vi "Main.vi"() -> ()   [LabVIEW 2019]
doc: "The myRIO Project template acquires acceleration data from the onboard accelerometer and displays the changes of acceleration values in a waveform chart."
uses:
  <vilib>/myRIO/Instrument Drivers/Onboard IO/PWM/typedefs/PWM Reference.ctl
  <vilib>/myRIO/Common/Instrument Driver Framework/Utilities/typedefs/myRIO Generic Hardware Reference.ctl
  <vilib>/myRIO/Common/Instrument Driver Framework/Utilities/typedefs/Hardware Version Enum.ctl
  <vilib>/myRIO/Common/Instrument Driver Framework/Utilities/typedefs/myRIO v1.0 Reference.ctl
  <vilib>/myRIO/Common/Instrument Driver Framework/Utilities/typedefs/Generic FPGA Reference.ctl
  <vilib>/myRIO/Common/Instrument Driver Framework/myRIO v1.0/PWM/typedefs/PWM Channels Enum.ctl
  <vilib>/myRIO/Instrument Drivers/Onboard IO/PWM/typedefs/PWM Configuration.ctl
  <vilib>/userDefined/High Color/nirio_resource_hc.ctl
  <vilib>/myRIO/Common/Instrument Driver Framework/Utilities/vis/Is FPGA Ref Available.vi
  <vilib>/myRIO/Common/Instrument Driver Framework/myRIO v1.0/PWM/vis/myRIO v1.1 Open PWM.vi
  <vilib>/myRIO/Instrument Drivers/Onboard IO/PWM/vis/Set Duty Cycle and Frequency.vi
  <vilib>/myRIO/Common/Instrument Driver Framework/Utilities/vis/Validate Channels.vi
  <vilib>/myRIO/Common/Instrument Driver Framework/myRIO v1.0/PWM/vis/myRIO v1.0 Reserve PWM.vi
  <vilib>/myRIO/Common/Instrument Driver Framework/myRIO v1.0/PWM/vis/myRIO v1.0 Build MUX Configuration PWM.vi
  <vilib>/myRIO/Common/Instrument Driver Framework/myRIO v1.0/Resource Manager/vis/myRIO v1.0 Reserve Channel List.vi
  <vilib>/myRIO/Common/Instrument Driver Framework/myRIO v1.0/Resource Manager/vis/myRIO v1.0 Create Configuration List.vi
  <vilib>/myRIO/Common/Instrument Driver Framework/myRIO v1.0/Resource Manager/vis/myRIO v1.0 Reserve Channel.vi
  <vilib>/myRIO/Common/Instrument Driver Framework/myRIO v1.0/Resource Manager/vis/myRIO v1.0 Unreserve Channel.vi
  <vilib>/myRIO/Common/Instrument Driver Framework/myRIO v1.0/Resource Manager/vis/myRIO v1.0 Build Mutex Name.vi
  <vilib>/Utility/VariantDataType/GetNumericInfo.vi
  <vilib>/Utility/error.llb/Error Cluster From Error Code.vi
  <vilib>/myRIO/Common/Instrument Driver Framework/myRIO v1.0/myRIO v1.1 Open.vi
  <vilib>/myRIO/Common/Instrument Driver Framework/Utilities/vis/IO Manager.vi
  <vilib>/myRIO/Common/Instrument Driver Framework/Utilities/vis/Configuration Manager.vi
  <vilib>/myRIO/Common/Instrument Driver Framework/myRIO v1.0/Resource Manager/vis/myRIO v1.0 Configure IO.vi
  <vilib>/myRIO/Common/Instrument Driver Framework/myRIO v1.0/myRIO v1.0 Close.vi
  <vilib>/myRIO/Common/Instrument Driver Framework/myRIO v1.0/PWM/vis/myRIO v1.0 Write PWM.vi
  <vilib>/myRIO/Express VI/Onboard IO/PWM/PWM Express VI.xnode
  <vilib>/myRIO/Instrument Drivers/Onboard IO/PWM/vis/myRIO PWM Open.xnode
  <vilib>/myRIO/Instrument Drivers/Onboard IO/PWM/PWM.lvlib
panel:
  in  "Numeric Control":i32
  in  "kruispunt verder":bool
  in  "hij mag weer verderrijden (na noodstop)":bool
  in  "noodstop":bool
  out "welk kruispunt":i32
  in  "Hoofdprogramma(einde)":bool
  out "de huidige afslag":string
  out "waardes van de reflectiesensor":dbl[](array[numeric])
  out "rechtermotor":dbl(knob) scale=0.0..10.0
  out "linkermotor":dbl(knob) scale=0.0..10.0
  in  "snelheidsverdeling":dbl(slide) scale=-5.0..5.0
  in  "snelheid":dbl(slide) scale=0.0..10.0
  in  "manual override?":bool
  in  "de afslagen":string[](array[string])
  # "links"
  # "rechts"
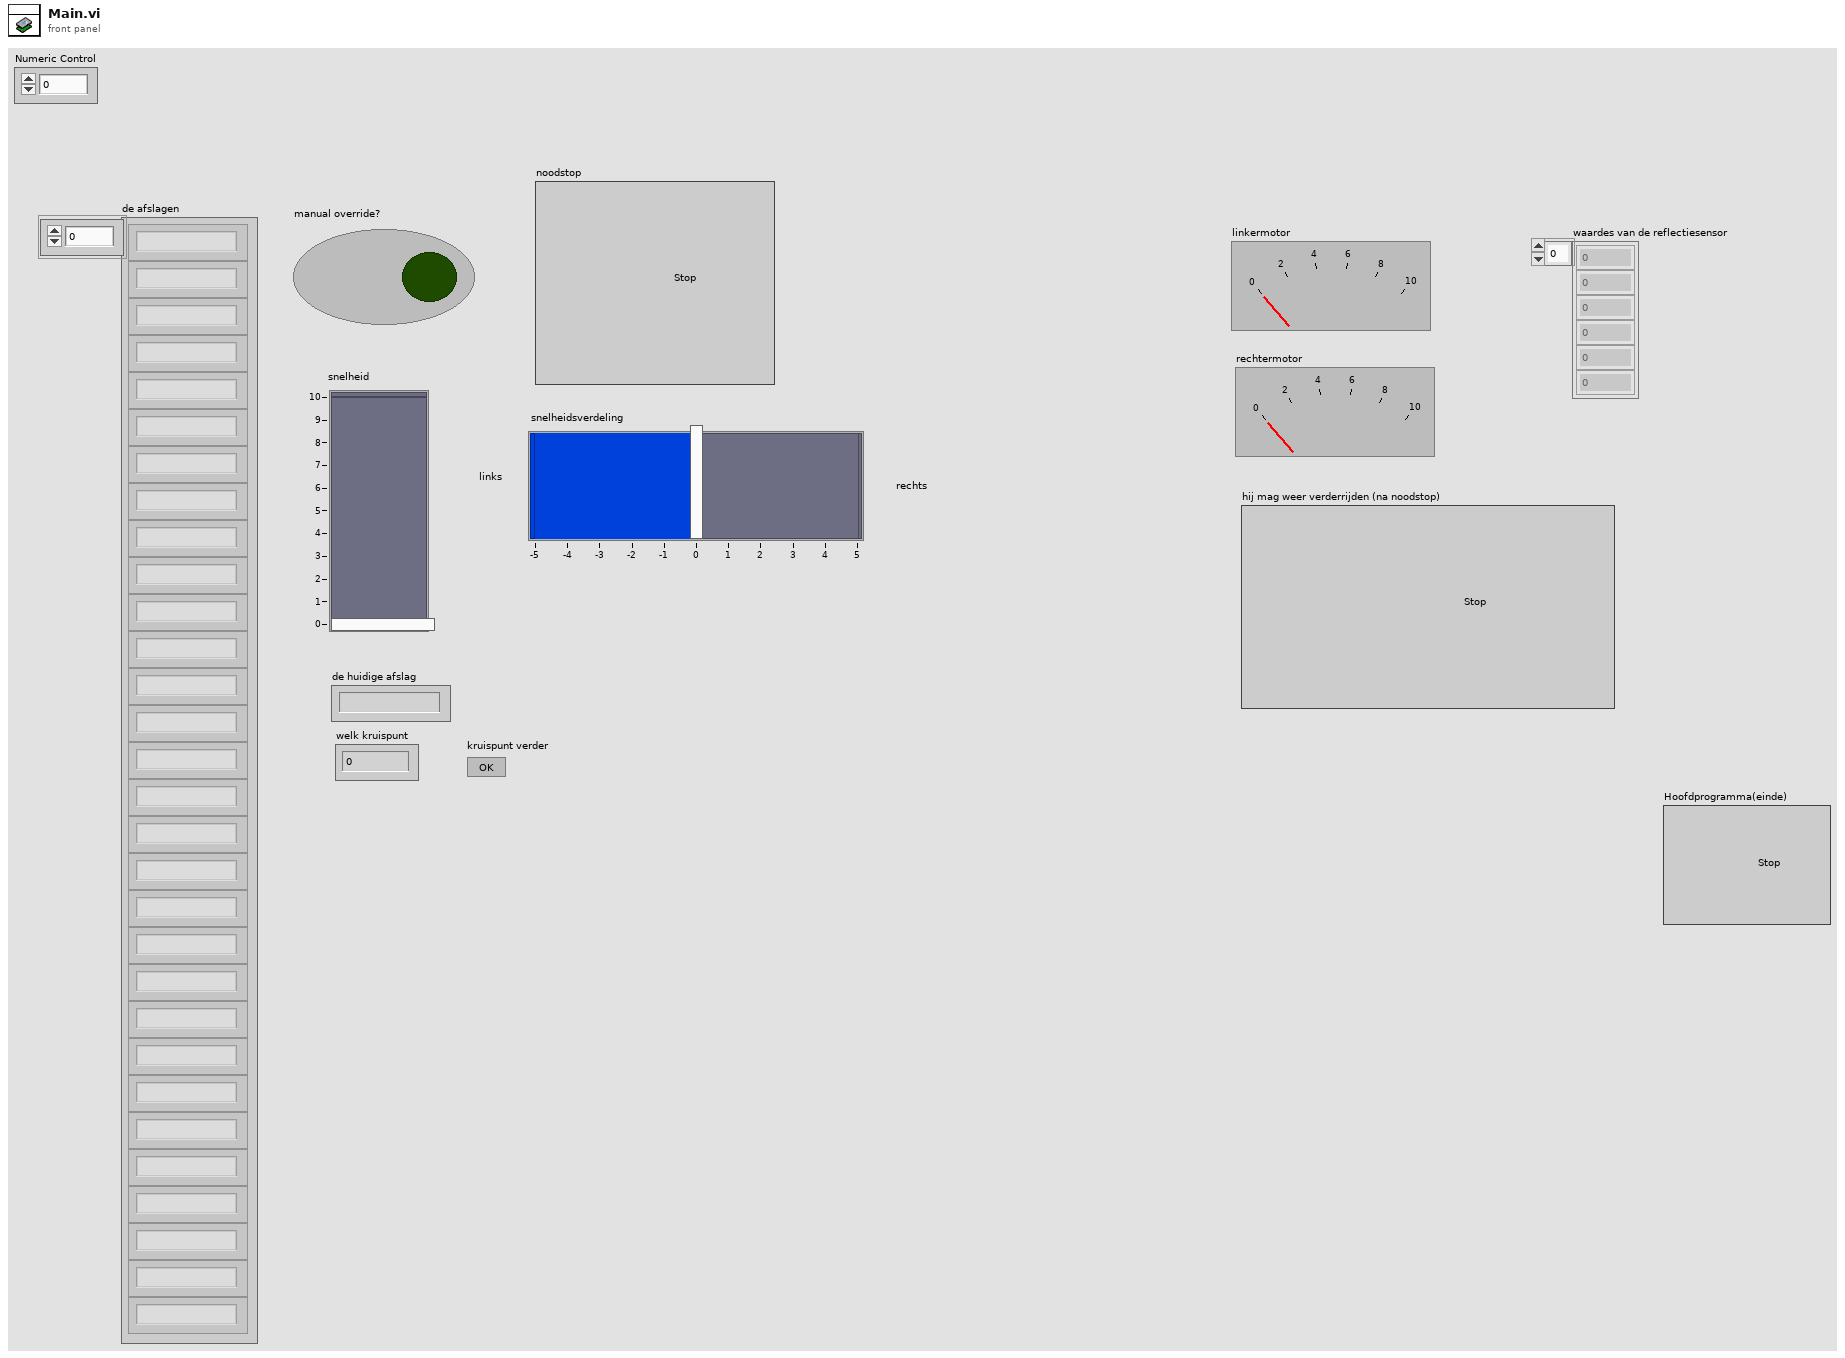
[diagram p1: front panel]
types:
  T1 = typedef "PWM.lvlib/PWM Reference.ctl" = cluster{"myRIO Reference":T2, "PWM Channels Enum":T6, "PWM Configuration":T7}
  T2 = typedef "myRIO Generic Hardware Reference.ctl" = cluster{"myRIO Model":T3, "myRIO Hardware Reference":T4}
  T3 = typedef "Hardware Version Enum.ctl" = enum16{"Unknown", "myRIO-1900", "myRIO-1950", "roboRIO", "NI ELVIS RIO CM", "ELVIS III"}
  T4 = typedef "myRIO v1.0 Reference.ctl" = cluster{"Generic FPGA Reference":T5, "Allow multiple opens":bool}
  T5 = typedef "Generic FPGA Reference.ctl" = refnum<k20>
  T6 = typedef "PWM Channels Enum.ctl" = enum16{"Not Connected", "C/PWM0", "C/PWM1", "A/PWM0", "A/PWM1", "A/PWM2", "A/PWM3", "A/PWM4", "A/PWM5", "A/PWM6", "A/PWM7", "A/PWM8", "A/PWM9", "A/PWM10", "A/PWM11", "A/PWM12", "A/PWM13", "A/PWM14", "A/PWM15", "A/PWM16", "A/PWM17", "A/PWM18", "A/PWM19", "B/PWM0", "B/PWM1", "B/PWM2", "B/PWM3", "B/PWM4", "B/PWM5", "B/PWM6", "B/PWM7", "B/PWM8", "B/PWM9", "B/PWM10", "B/PWM11", "B/PWM12", "B/PWM13", "B/PWM14", "B/PWM15", "B/PWM16", "B/PWM17", "B/PWM18", "B/PWM19", "PWM/PWM0", "PWM/PWM1", "PWM/PWM2", "PWM/PWM3", "PWM/PWM4", "PWM/PWM5", "PWM/PWM6", "PWM/PWM7", "PWM/PWM8", "PWM/PWM9"}
  T7 = typedef "PWM.lvlib/PWM Configuration.ctl" = cluster{"Frequency":dbl, "Duty Cycle":dbl}
  T8 = typedef "nirio_resource_hc.ctl" = tag
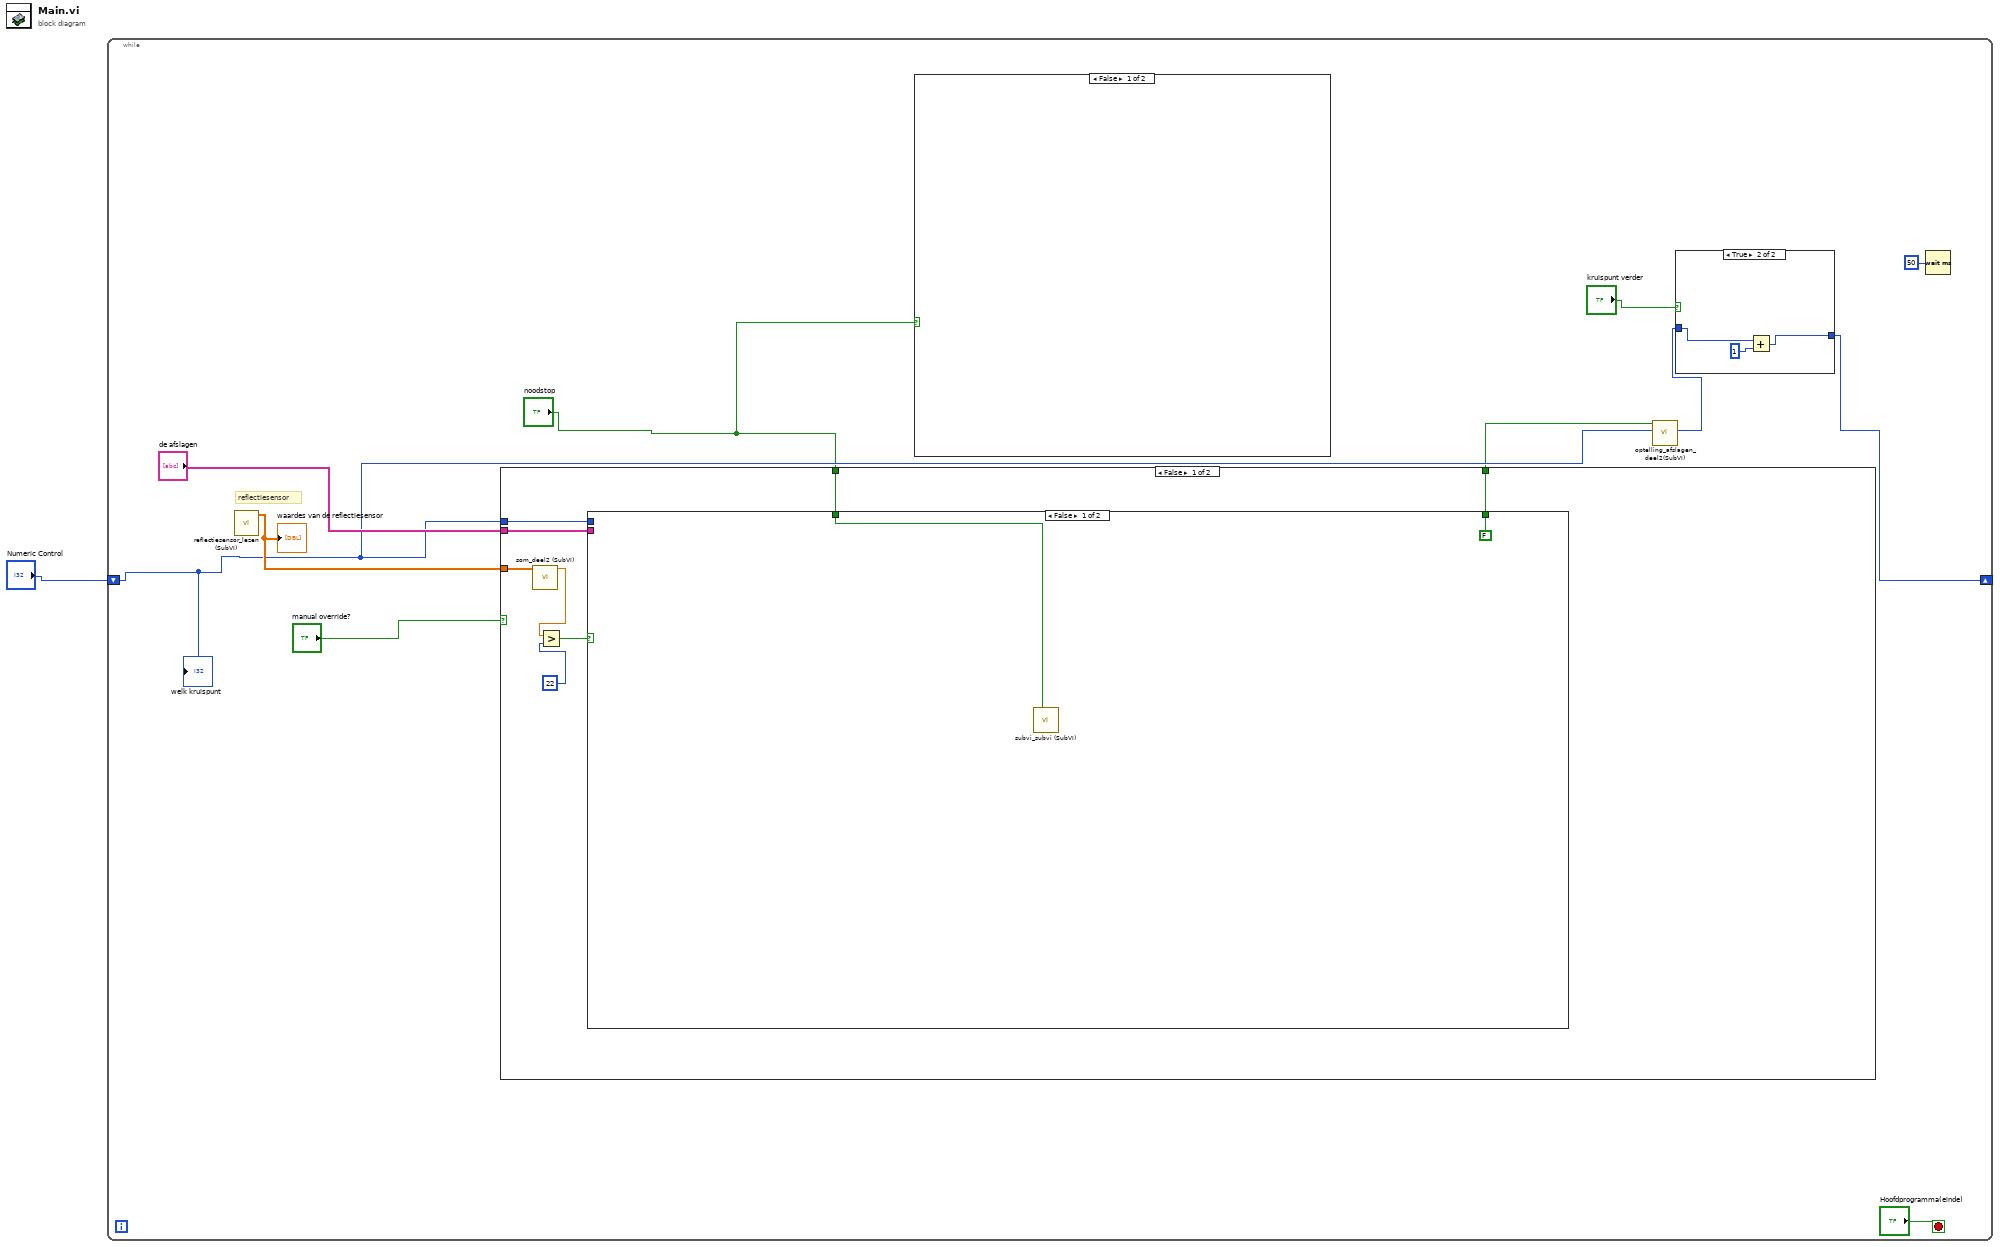
[diagram p0: block diagram]
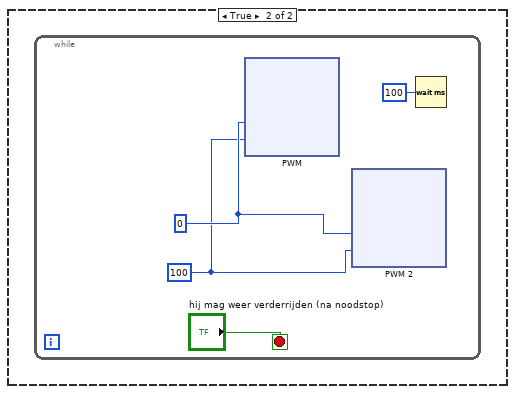
[diagram p3: hidden frame]
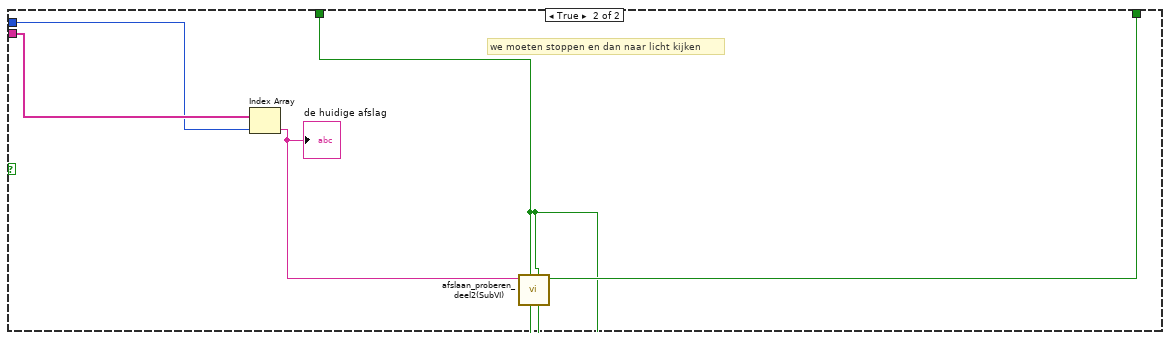
[diagram p4: hidden frame]
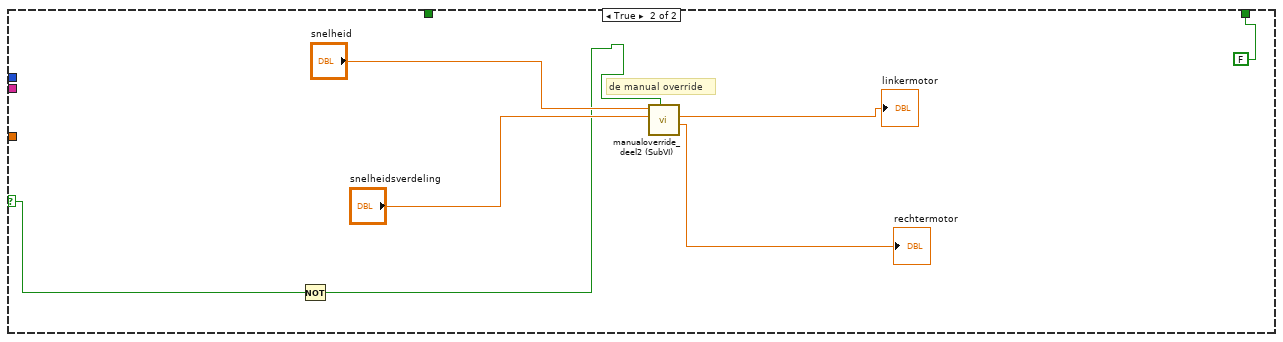
[diagram p5: hidden frame]
diagram:
  n1 = while {
    shift-right: [w4] -> _
    shift-left: "Numeric Control" -> [w9]
    stop <- "Hoofdprogramma(einde)" stop-if-true
    # "reflectiesensor"
    n2 = call "reflectiesensor_lezen (SubVI).vi"() -> ("Values"=w11:dbl[])  [unwired: 11 in]
    "waardes van de reflectiesensor" <- w11
    n3 = case shown="False" "manual override?" {
      selector: "manual override?" -> [_ w107]
      tunnel: w11 -> [w98 _]
      tunnel: "de afslagen" -> [w97 _]
      tunnel: w9 -> [w96 _]
      tunnel: [w92 FALSE] -> w8
      tunnel: "noodstop" -> [w91 _]
      frame False {
        n4 = call "som_deel2 (SubVI).vi"("array"=w98) -> ("x+y"=w95:dbl)  [unwired: 10 in]
        n5 = Greater?(x=w95, y=22) -> (0:w93:bool)
        n6 = case shown="False" w93 {
          tunnel: w97 -> [_ w105]
          tunnel: w96 -> [_ w104]
          tunnel: [FALSE w102] -> w92
          tunnel: w91 -> [w99 w101]
          frame False {
            n7 = call "subvi_subvi (SubVI).vi"("stop"=w99) -> ()  [unwired: 11 in]
          }
          frame True {
            # "we moeten stoppen en dan naar licht kijken"
            n8 = Index Array(array=w105, index=w104) -> (element=w103:string)
            "de huidige afslag" <- w103
            n9 = call "afslaan_proberen_deel2(SubVI).vi"("stop 3"=w101, "stop"=w101, "stop 2"=w101, "universele stop"=w101, "element"=w103) -> ("OK Button 2"=w102:bool)  [unwired: 6 in]
          }
        }
      }
      frame True {
        # "de manual override"
        n10 = Not(x=w107) -> (.not. x?=w106:bool)
        n11 = call "manualoverride_deel2 (SubVI).vi"("stop"=w106, "snelheidsverdeling"="snelheidsverdeling", "snelheid"="snelheid") -> ("rechtermotor na"=→"rechtermotor":dbl, "linkermotor na"=→"linkermotor":dbl)  [unwired: 7 in]
      }
    }
    n12 = case shown="False" "noodstop" {
      frame False {
      }
      frame True {
        n13 = while {
          stop <- "hij mag weer verderrijden (na noodstop)" stop-if-true
          w17 = 100
          w18 = 0
          n14 = xnode "PWM"("Duty Cycle"=w18, "Frequency [Hz]"=w17) -> ()  [unwired: 1 in, 1 out]
          n15 = xnode "PWM 2"("Duty Cycle"=w18, "Frequency [Hz]"=w17) -> ()  [unwired: 1 in, 1 out]
          n16 = Wait (ms)(milliseconds to wait=u32 100) -> ()  [unwired: 1 out]
        }
      }
    }
    n17 = call "optelling_afslagen_deel2(SubVI).vi"("Numeric"=w9, "OK Button"=w8) -> ("Numeric 2"=w5:i32)  [unwired: 9 in]
    n18 = case shown="True" "kruispunt verder" {
      tunnel: w5 -> [w13 w16]
      tunnel: [w13 w14] -> w4
      frame False {
      }
      frame True {
        n19 = Add(x=w16, y=1) -> (x+y=w14:i32)
      }
    }
    n20 = Wait (ms)(milliseconds to wait=u32 50) -> ()  [unwired: 1 out]
    "welk kruispunt" <- w9
  }
